vi "Main.vi"(11 "Module Admin":refnum<class "Delacor_lib_QMH_Module Admin.lvclass">) -> ()   [LabVIEW 2020, in "General UI.lvlib"]
doc: "This template is based off of the Queued Message Handler design pattern and the Queued Message Handler project template that ships with LabVIEW.\n\nThe main difference is that the queue is private to this module and communication between modules is performed via Broadcast and Request events.\n\nRequest events are wrapped in public API methods and are handled in the Event Handling Loop (EHL) of this VI. Any module can register for Broadcast events sent by this module. The EHL generates messages based on user interface actions.\n\nThe Message Handling Loop (MHL) processes messages generated by the EHL, or by other messages. The messages are string values, so new messages can be added easily to the Message Cases case structure in the MHL. Each message cluster can also provide an optional value for Message Data, which is a variant that can be converted to whatever message-specific data is required.\n_____\nBased on Delacor QMH Project Template 5.0.0.82."
uses:
  General UI.lvlib
  <vilib>/Delacor/Delacor QMH/Libraries/Module Admin_class/Delacor_lib_QMH_Module Admin.lvclass
  Module Data--cluster.ctl
  Stop Argument--cluster.ctl
  <vilib>/Delacor/Delacor QMH/Libraries/Message Queue_class/Delacor_lib_QMH_Message Queue.lvclass/Delacor_lib_QMH_Message Queue.ctl
  <vilib>/Delacor/Delacor QMH/Libraries/Module Admin_class/Delacor_lib_QMH_Module Admin.lvclass/Delacor_lib_QMH_Module Admin.ctl
  <vilib>/Delacor/Delacor QMH/Libraries/Message Queue_class/Delacor_lib_QMH_Enqueue Message (Single).vi
  <vilib>/Delacor/Delacor QMH/Libraries/Module Admin_class/Delacor_lib_QMH_Get External Launch.vi
  <vilib>/Utility/error.llb/Error Cluster From Error Code.vi
  <vilib>/ErrorRing/Error Ring.xnode
  <vilib>/Delacor/Delacor QMH/Libraries/Message Queue_class/Delacor_lib_QMH_Message Queue.lvclass
  Money Control Pane/Money Control Pane.lvlib
  Product Selecting Pane/Product Selecting Pane.lvlib
  Message Pane/Message Pane.lvlib
panel:
  out "error out":errorcluster
  in  "Exit":bool
  in  "Settings":bool
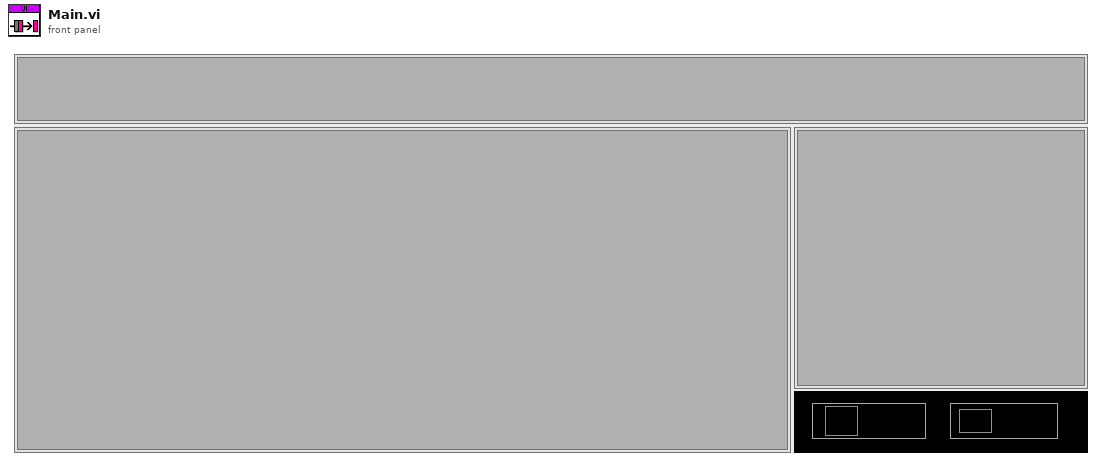
[diagram p1: front panel]
types:
  T1 = typedef "General UI.lvlib/Request Events--cluster.ctl" = cluster{"Stop Module":refnum<user-event>, "Show Panel":refnum<user-event>, "Hide Panel":refnum<user-event>, "Get Module Execution Status":refnum<user-event>, "Show Diagram":refnum<user-event>}
  T2 = typedef "Money Control Pane.lvlib/Broadcast Events--cluster.ctl" = cluster{"Module Did Init":refnum<user-event>, "Status Updated":refnum<user-event>, "Error Reported":refnum<user-event>, "Module Did Stop":refnum<user-event>, "Update Module Execution Status":refnum<user-event>}
  T3 = typedef "Product Selecting Pane.lvlib/Broadcast Events--cluster.ctl" = cluster{"Module Did Init":refnum<user-event>, "Status Updated":refnum<user-event>, "Error Reported":refnum<user-event>, "Module Did Stop":refnum<user-event>, "Update Module Execution Status":refnum<user-event>}
  T4 = typedef "Message Pane.lvlib/Broadcast Events--cluster.ctl" = cluster{"Module Did Init":refnum<user-event>, "Status Updated":refnum<user-event>, "Error Reported":refnum<user-event>, "Module Did Stop":refnum<user-event>, "Update Module Execution Status":refnum<user-event>}
  T5 = typedef "General UI.lvlib/Module Data--cluster.ctl" = cluster{"Status":string}
  T6 = enum32{"invalid lock state", "Not Locked", "Locked (No Password)", "Password-protected"}
  T7 = typedef "General UI.lvlib/Stop Argument--cluster.ctl" = cluster{"Origin":string, "Exit via Stop Module Req?":bool, "Wait for Module to stop?":bool}
  T8 = enum32{"Invalid", "Standard", "Closed", "Hidden", "Minimized", "Maximized"}
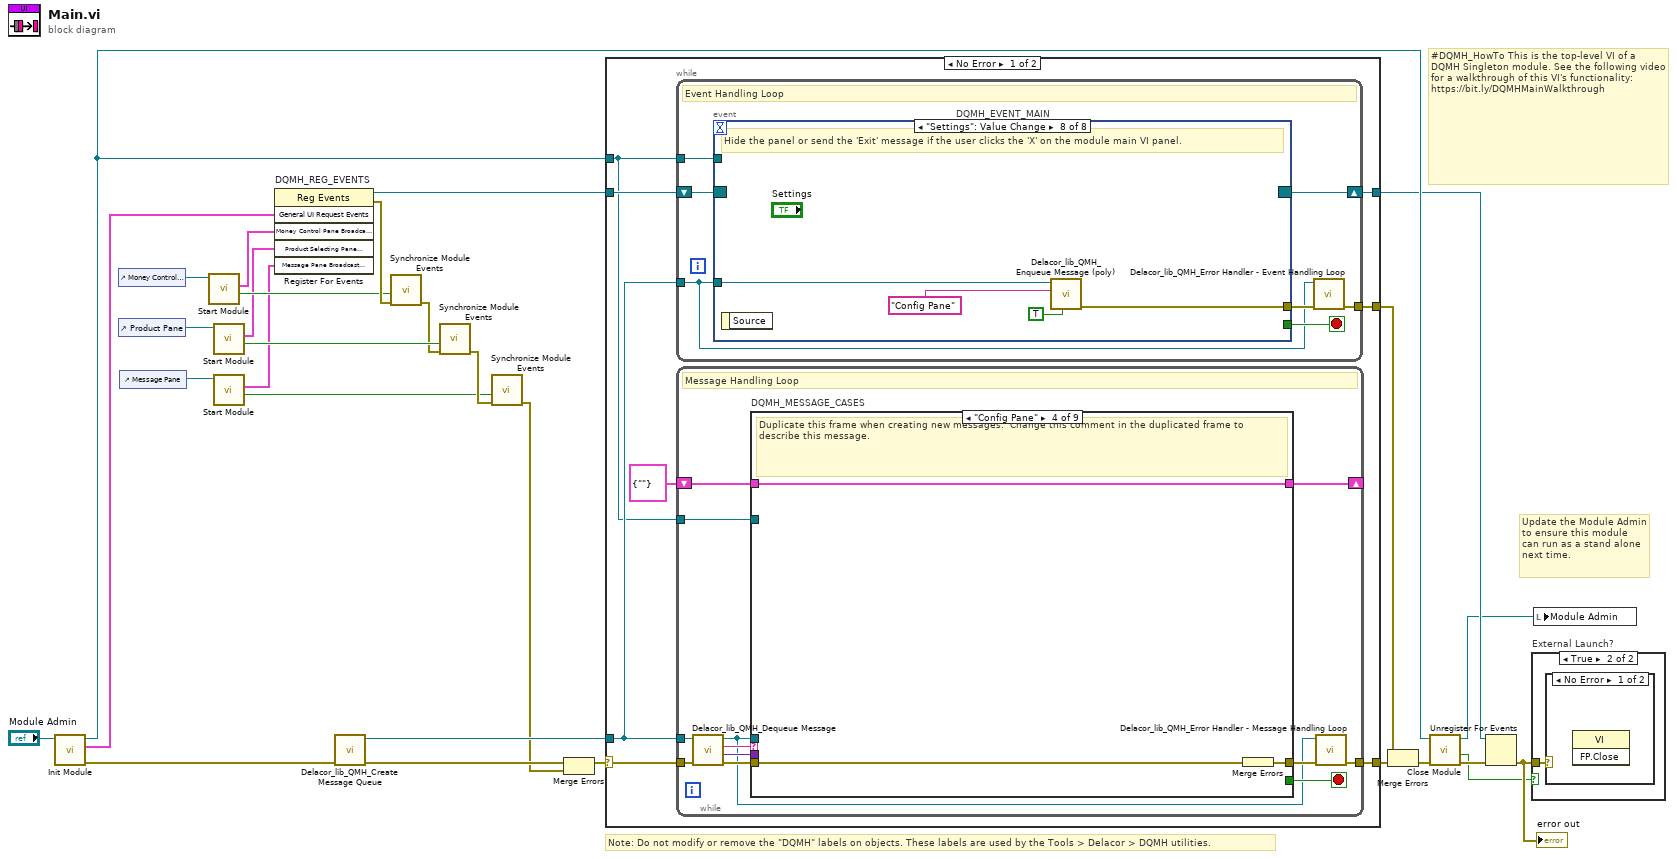
[diagram p0: block diagram]
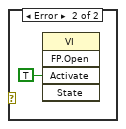
[diagram p3: hidden frame]
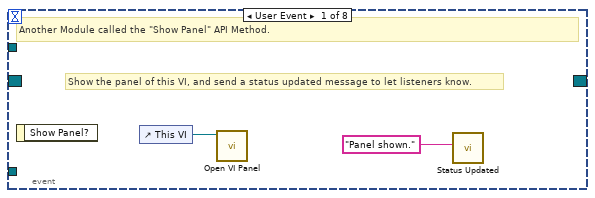
[diagram p4: hidden frame]
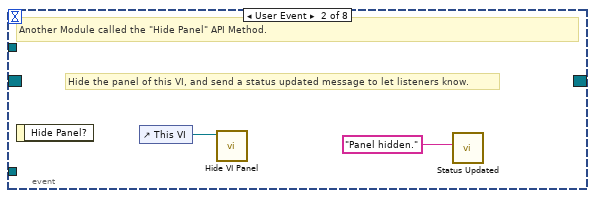
[diagram p5: hidden frame]
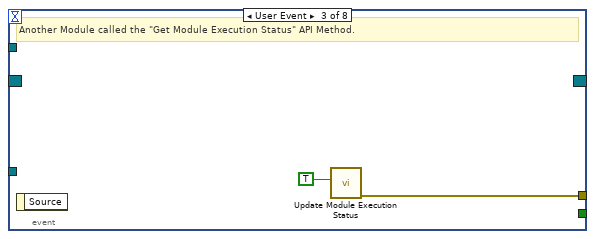
[diagram p6: hidden frame]
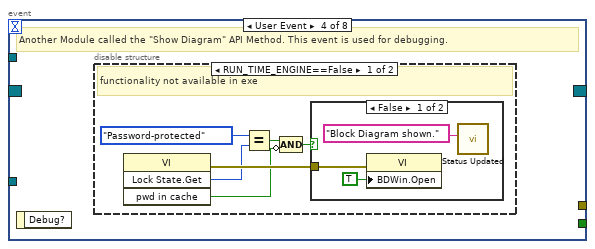
[diagram p7: hidden frame]
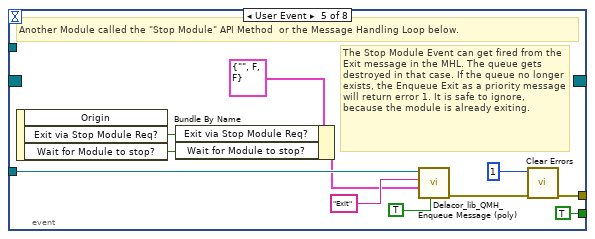
[diagram p10: hidden frame]
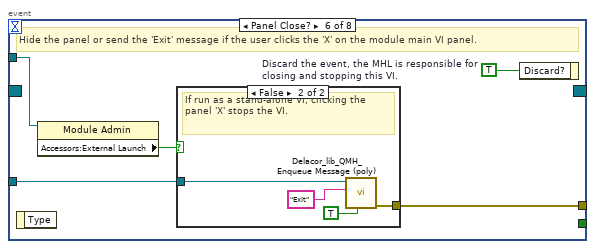
[diagram p11: hidden frame]
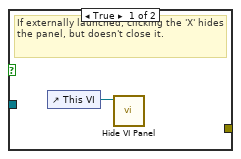
[diagram p12: hidden frame]
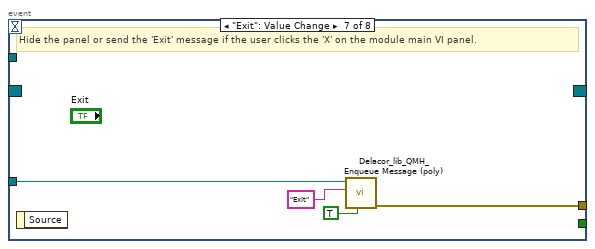
[diagram p13: hidden frame]
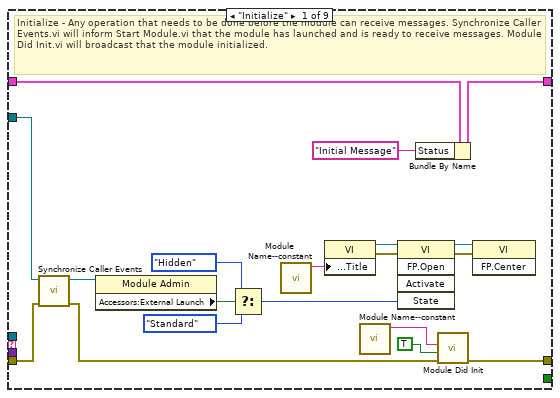
[diagram p14: hidden frame]
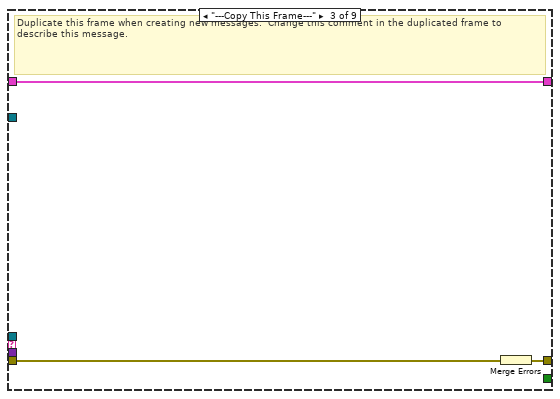
[diagram p16: hidden frame]
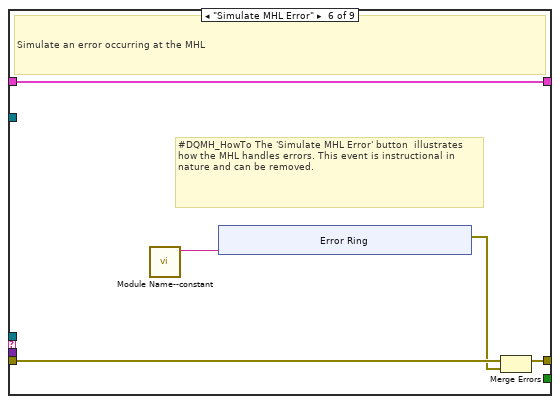
[diagram p18: hidden frame]
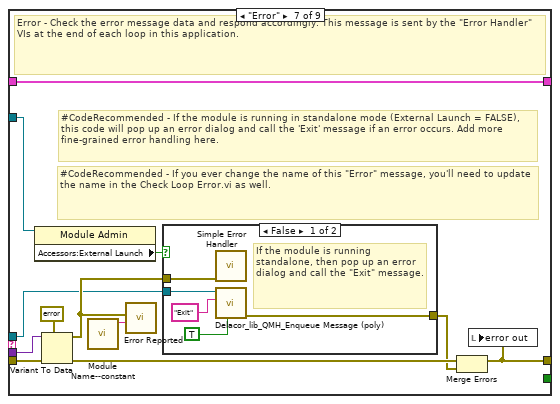
[diagram p19: hidden frame]
diagram:
  # "#DQMH_HowTo This is the top-level VI of a DQMH Singleton module. See the following video for a walkthrough of this VI's functionality: https://bit.ly/DQMHMainWalkthrough"
  # "Note: Do not modify or remove the \"DQMH\" labels on objects. These labels are used by the Tools > Delacor > DQMH utilities."
  # "Update the Module Admin to ensure this module can run as a stand alone next time."
  n1 = call "Init Module.vi"("Singleton Module Admin in"="Module Admin") -> ("error out"=w28:errorcluster, "General UI Request Events"=w18:T1, "Singleton Module Admin out"=w21:refnum<class "Delacor_lib_QMH_Module Admin.lvclass">)  [unwired: 8 in]
  n2 = control-ref of="Money Control Pane"() -> (w13:refnum<vi>)
  n3 = control-ref of="Product Pane"() -> (w9:refnum<vi>)
  n4 = control-ref of="Message Pane"() -> (w5:refnum<vi>)
  n5 = call "Start Module.vi"("MCP Sub Panel"=w13) -> ("Wait for Event Sync?"=w10:bool, "Money Control Pane Broadcast Events"=w12:T2)  [unwired: 7 in, 2 out]
  n6 = call "Start Module.vi"("Sub Panel"=w9) -> ("Wait for Event Sync?"=w8:bool, "Product Selecting Pane Broadcast Events"=w7:T3)  [unwired: 7 in, 2 out]
  n7 = call "Start Module.vi"("Sub Panel"=w5) -> ("Wait for Event Sync?"=w2:bool, "Message Pane Broadcast Events"=w1:T4)  [unwired: 7 in, 2 out]
  n8 = register-events "DQMH_REG_EVENTS"(w18, w12, w7, w1) -> (reference out=w19:refnum<event-registration>, error out=w11:errorcluster)  [unwired: 2 in]
  n9 = call <vilib>:"Delacor_lib_QMH_Create Message Queue.vi"("error in (no error)"=w28) -> ("error out"=w23:errorcluster, "Message Queue"=w17:refnum<class "Delacor_lib_QMH_Message Queue.lvclass">)  [unwired: 9 in]
  n10 = call "Synchronize Module Events.vi"("error in (no error)"=w11, "Wait for Event Sync?"=w10) -> ("error out"=w6:errorcluster)  [unwired: 9 in]
  n11 = call "Synchronize Module Events.vi"("error in (no error)"=w6, "Wait for Event Sync?"=w8) -> ("error out"=w4:errorcluster)  [unwired: 9 in]
  n12 = call "Synchronize Module Events.vi"("error in (no error)"=w4, "Wait for Event Sync?"=w2) -> ("error out"=w3:errorcluster)  [unwired: 9 in]
  n13 = Merge Errors(w23, w3) -> (w22:errorcluster)
  n14 = case shown="No Error" w22 {
    selector: w22 -> [w35 w190]
    tunnel: [w37 w189] -> w29
    tunnel: [w34 w195] -> w20
    tunnel: w19 -> [w32 w195]
    tunnel: w17 -> [w31 w188]
    tunnel: [w36 _] -> w26
    tunnel: w21 -> [w30 w191]
    frame No Error {
      n15 = while {
        tunnel: w31 -> [w38]
        shift-right: [w41] -> w34
        shift-left: w32 -> [w42]
        tunnel: [w43] -> w36
        tunnel: w30 -> [w39]
        stop <- w40 stop-if-true
        # "Event Handling Loop"
        n16 = event "DQMH_EVENT_MAIN" shown="[7] \"Settings\": Value Change" {
          selector: w42 -> [_ _ _ _ _ _ _ _]
          dyn-events: [_ _ _ _ _ _ _ _] -> w41
          timeout: _ -> [_ _ _ _ _ _ _ _]
          tunnel: [_ _ _ _ TRUE ("Discard?") _ _ _] -> w40
          tunnel: w38 -> [_ _ _ _ w66 w73 w83 w87]
          tunnel: [_ _ w50 _ w69 w75 w84 w88] -> w44
          tunnel: w39 -> [_ _ _ _ _ w72 _ _]
          event User Event {
            # "Show the panel of this VI, and send a status updated message to let listeners know."
            # "Another Module called the \"Show Panel\" API Method."
            n17 = event-data() -> ()  [unwired: 1 in, 1 out]
            n18 = control-ref of="This VI"() -> (w46:refnum<vi>)
            n19 = call "Open VI Panel.vi"("VI"=w46) -> ()  [unwired: 10 in, 1 out]
            n20 = call "Status Updated.vi"("Status"="Panel shown." ("format string")) -> ()  [unwired: 10 in, 1 out]
          }
          event User Event {
            # "Hide the panel of this VI, and send a status updated message to let listeners know."
            # "Another Module called the \"Hide Panel\" API Method."
            n21 = event-data() -> ()  [unwired: 1 in, 1 out]
            n22 = control-ref of="This VI"() -> (w48:refnum<vi>)
            n23 = call "Hide VI Panel.vi"("VI"=w48) -> ()  [unwired: 10 in, 1 out]
            n24 = call "Status Updated.vi"("Status"="Panel hidden." ("format string")) -> ()  [unwired: 10 in, 1 out]
          }
          event User Event {
            # "Another Module called the \"Get Module Execution Status\" API Method."
            n25 = event-data() -> ()  [unwired: 1 in, 1 out]
            n26 = call "Update Module Execution Status.vi"("Running?"=TRUE) -> ("error out"=w50:errorcluster)  [unwired: 10 in]
          }
          event User Event {
            # "Another Module called the \"Show Diagram\" API Method. This event is used for debugging."
            n27 = event-data() -> ()  [unwired: 1 in, 1 out]
            n28 = disable-structure shown="RUN_TIME_ENGINE==False" {
              frame condition #0 (active) {
                # "functionality not available in exe"
                n29 = invoke class="VI" method="Lock State.Get"() -> (error out=w56:errorcluster, "Get Lock State"=w55:T6, "pwd in cache"=w52:bool)  [unwired: 4 in, 1 out]
                n30 = Equal?(x=T6."Password-protected", y=w55) -> (x = y?=w53:bool)
                n31 = Compound Arithmetic op=AND(w53, invert w52) -> (w51:bool)
                n32 = case shown="False" w51 {
                  tunnel: w56 -> [w59 _]
                  frame False {
                    n33 = property class="VI"(error in=w59, "BDWin.Open"=TRUE ("Block Diagram Window:Open")) -> ()  [unwired: 1 in, 2 out]
                    n34 = call "Status Updated.vi"("Status"="Block Diagram shown." ("format string")) -> ()  [unwired: 10 in, 1 out]
                  }
                  frame True {
                    # "Password-protected VI, and the password is not in the cache. Do not show the diagram."
                  }
                }
              }
              frame condition #1 {
              }
            }
          }
          event User Event {
            # "The Stop Module Event can get fired from the Exit message in the MHL. The queue gets destroyed in that case. If the queue no longer exists, the Enqueue Exit as a priority message will return error 1. It is safe to ignore, because the module is already exiting."
            # "Another Module called the \"Stop Module\" API Method  or the Message Handling Loop below."
            n35 = event-data() -> ("Exit via Stop Module Req?"=w62:bool, "Wait for Module to stop?"=w61:bool)  [unwired: 1 in, 1 out]
            n36 = Bundle By Name(cluster=T7 {"Origin"="", "Exit via Stop Module Req?"=FALSE, "Wait for Module to stop?"=FALSE} ("Stop Argument"), "Exit via Stop Module Req?"=w62, "Wait for Module to stop?"=w61) -> (w60:T7)
            n37 = call-poly <vilib>:"Delacor_lib_QMH_Enqueue Message (poly).vi"("Priority Message? (F)"=TRUE, "Message Data"=w60, "Message"="Exit", "Message Queue in"=w66) -> ("error out"=w70:errorcluster)  [unwired: 6 in, 1 out]
            n38 = call <vilib>:"Clear Errors.vi"("error in (no error)"=w70, "specific error code to clear (0: all)"=1) -> ("error out"=w69:errorcluster)  [unwired: 4 in, 1 out]
          }
          event Panel Close? {
            w74 = TRUE  # Discard the event, the MHL is responsible for closing and stopping this VI.
            # "Hide the panel or send the 'Exit' message if the user clicks the 'X' on the module main VI panel."
            n39 = event-data() -> ()  [unwired: 1 in, 1 out]
            n40 = property class="Module Admin"(reference=w72) -> ("Accessors:External Launch"=w71:bool)  [unwired: 1 in, 2 out]
            n41 = case shown="False" w71 {
              tunnel: w73 -> [_ w79]
              tunnel: [_ w80] -> w75
              frame True {
                # "If externally launched, clicking the 'X' hides the panel, but doesn't close it."
                n42 = control-ref of="This VI"() -> (w76:refnum<vi>)
                n43 = call "Hide VI Panel.vi"("VI"=w76) -> ()  [unwired: 10 in, 1 out]
              }
              frame False {
                # "If run as a stand-alone VI, clicking the panel 'X' stops the VI."
                n44 = call-poly <vilib>:"Delacor_lib_QMH_Enqueue Message (poly).vi"("Priority Message? (F)"=TRUE, "Message"="Exit", "Message Queue in"=w79) -> ("error out"=w80:errorcluster)  [unwired: 7 in, 1 out]
              }
            }
            n45 = event-data("Discard?"=w74) -> ()  [unwired: 1 in, 1 out]
          }
          event "Exit": Value Change {
            # "Hide the panel or send the 'Exit' message if the user clicks the 'X' on the module main VI panel."
            n46 = event-data() -> ()  [unwired: 1 in, 1 out]
            n47 = call-poly <vilib>:"Delacor_lib_QMH_Enqueue Message (poly).vi"("Priority Message? (F)"=TRUE, "Message"="Exit", "Message Queue in"=w83) -> ("error out"=w84:errorcluster)  [unwired: 7 in, 1 out]
          }
          event "Settings": Value Change {
            # "Hide the panel or send the 'Exit' message if the user clicks the 'X' on the module main VI panel."
            n48 = event-data() -> ()  [unwired: 1 in, 1 out]
            n49 = call-poly <vilib>:"Delacor_lib_QMH_Enqueue Message (poly).vi"("Priority Message? (F)"=TRUE, "Message"="Config Pane", "Message Queue in"=w87) -> ("error out"=w88:errorcluster)  [unwired: 7 in, 1 out]
          }
        }
        n50 = call-dynamic "Delacor_lib_QMH_Error Handler - Event Handling Loop.vi"("error in (no error)"=w44, "Message Queue in"=w38) -> ("dup error in"=w43:errorcluster)  [unwired: 8 in, 1 out]
      }
      n51 = while {
        tunnel: w31 -> [w91]
        shift-right: [w95] -> _
        shift-left: T5 {"Status"=""} ("Data Cluster") -> [w96]
        tunnel: w35 -> [w99]
        tunnel: [w97] -> w37
        tunnel: w30 -> [w89]
        stop <- w94 stop-if-true
        # "Message Handling Loop"
        n52 = call-dynamic "Delacor_lib_QMH_Dequeue Message.vi"("error in (no error)"=w99, "Message Queue in"=w91) -> ("error out"=w98:errorcluster, "Message Data"=w92:variant, "Message"=w93:string, "Message Queue out"=w90:refnum<class "Delacor_lib_QMH_Message Queue.lvclass">)  [unwired: 6 in]
        n53 = case "DQMH_MESSAGE_CASES" shown="\"Config Pane\"" w93 {
          selector: w93 -> [_ _ _ _ _ _ _ _ w175]
          tunnel: w90 -> [_ _ _ _ _ _ w145 w167 _]
          tunnel: w98 -> [w117 w121 w124 w127 w129 w134 w152 w173 w177]
          tunnel: [w115 w121 w123 w126 w129 w133 w148 w170 w178] -> w100
          tunnel: w96 -> [w106 w120 w122 w125 w128 w131 w147 w166 w176]
          tunnel: [w105 w120 w122 w125 w128 w131 w147 w166 w176] -> w95
          tunnel: [_ _ _ _ _ _ _ w165 _] -> w94
          tunnel: w92 -> [_ _ _ _ _ _ w146 w164 _]
          tunnel: w89 -> [w107 _ _ _ _ _ w144 w159 _]
          frame "Initialize" {
            # "Initialize - Any operation that needs to be done before the module can receive messages. Synchronize Caller Events.vi will inform Start Module.vi that the module has launched and is ready to receive messages. Module Did Init.vi will broadcast that the module initialized."
            n54 = call "Synchronize Caller Events.vi"("error in (no error)"=w117, "Singleton Module Admin in"=w107) -> ("error out"=w116:errorcluster, "Singleton Module Admin out"=w102:refnum<class "Delacor_lib_QMH_Module Admin.lvclass">)  [unwired: 8 in]
            n55 = property class="Module Admin"(reference=w102) -> ("Accessors:External Launch"=w111:bool)  [unwired: 1 in, 2 out]
            n56 = Select(t=T8."Hidden" ("State"), s=w111, f=T8."Standard" ("State")) -> (s? t:f=w108:T8)
            n57 = call "Module Name--constant.vi"() -> ("Module Name"=w114:string)  [unwired: 11 in]
            n58 = property class="VI"("Front Panel.Title"=w114) -> (reference out=w113:refnum<vi>, error out=w119:errorcluster)  [unwired: 2 in]
            n59 = call "Module Name--constant.vi"() -> ("Module Name"=w103:string)  [unwired: 11 in]
            n60 = invoke class="VI" method="FP.Open"(reference=w113, error in=w119, "State"=w108) -> (reference out=w112:refnum<vi>, error out=w118:errorcluster)  [unwired: 2 in, 3 out]
            n61 = Bundle By Name(cluster=w106, "Status"="Initial Message" ("Initial Message")) -> (w105:T5)
            n62 = call "Module Did Init.vi"("error in (no error)"=w116, "Initialized?"=TRUE, "Origin"=w103) -> ("error out"=w115:errorcluster)  [unwired: 8 in]
            n63 = invoke class="VI" method="FP.Center"(reference=w112, error in=w118) -> ()  [unwired: 1 in, 3 out]
          }
          frame "--- Module Specific ---" {
            # "Separator -- The following cases handle messages specific to this Module."
          }
          frame "---Copy This Frame---" {
            # "Duplicate this frame when creating new messages.  Change this comment in the duplicated frame to describe this message."
            n64 = Merge Errors(w124) -> (w123:errorcluster)
          }
          frame "Config Pane" {
            # "Duplicate this frame when creating new messages.  Change this comment in the duplicated frame to describe this message."
            n65 = Merge Errors(w127) -> (w126:errorcluster)
          }
          frame "--- Exit and Error Handling---" {
            # "Separator - The following cases handle errors and exit messages."
          }
          frame "Simulate MHL Error" {
            # "#DQMH_HowTo The 'Simulate MHL Error' button  illustrates how the MHL handles errors. This event is instructional in nature and can be removed."
            # "Simulate an error occurring at the MHL"
            n66 = call "Module Name--constant.vi"() -> ("Module Name"=w130:string)  [unwired: 11 in]
            n67 = xnode "Error Ring"("parameter 0"=w130) -> ("error out"=w132:errorcluster)
            n68 = Merge Errors(w134, w132) -> (w133:errorcluster)
          }
          frame "Error" {
            # "#CodeRecommended - If you ever change the name of this \"Error\" message, you'll need to update the name in the Check Loop Error.vi as well."
            # "#CodeRecommended - If the module is running in standalone mode (External Launch = FALSE), this code will pop up an error dialog and call the 'Exit' message if an error occurs. Add more fine-grained error handling here."
            # "Error - Check the error message data and respond accordingly. This message is sent by the \"Error Handler\" VIs at the end of each loop in this application."
            n69 = property class="Module Admin"(reference=w144) -> ("Accessors:External Launch"=w143:bool)  [unwired: 1 in, 2 out]
            n70 = Variant To Data(error in=w152, type=errorcluster {"status"=FALSE, "code"=0, "source"=""} ("error constant"), Variant=w146) -> (data=w153:errorcluster, error out=w150:errorcluster)
            n71 = call "Module Name--constant.vi"() -> ("Module Name"=w142:string)  [unwired: 11 in]
            n72 = call "Error Reported.vi"("Additional Information"=w142, "Error"=w153) -> ()  [unwired: 9 in, 1 out]
            n73 = case shown="False" w143 {
              tunnel: [w158 _] -> w149
              tunnel: w145 -> [w156 _]
              tunnel: w153 -> [w157 _]
              frame False {
                # "If the module is running standalone, then pop up an error dialog and call the \"Exit\" message."
                n74 = call <vilib>:"Simple Error Handler.vi"("error in (no error)"=w157) -> ()  [unwired: 4 in, 5 out]
                n75 = call-poly <vilib>:"Delacor_lib_QMH_Enqueue Message (poly).vi"("Priority Message? (F)"=TRUE, "Message"="Exit", "Message Queue in"=w156) -> ("error out"=w158:errorcluster)  [unwired: 7 in, 1 out]
              }
              frame True {
                # "If the module was launched externally, calling the Error Reported broadcast VI is the only action performed by the \"Error\" message. The module's caller can then process the error appropriately."
              }
            }
            n76 = Merge Errors(w150, w149) -> (w148:errorcluster)
            n77 = local write "error out"(w148) -> ()
          }
          frame "Exit" {
            w163 = 91  # 91: not all Exit messages will have an argument
            w165 = TRUE  # Stop the VI
            # "Release the message queue reference"
            # "#CodeNeeded - Add any required cleanup code here"
            # "Exit - Exit the application."
            n78 = Variant To Data(error in=w173, type=T7 {"Origin"="", "Exit via Stop Module Req?"=FALSE, "Wait for Module to stop?"=FALSE} ("Stop Argument"), Variant=w164) -> (data=w161:T7, error out=w169:errorcluster)
            n79 = call <vilib>:"Clear Errors.vi"("error in (no error)"=w169, "specific error code to clear (0: all)"=w163) -> ("error out"=w172:errorcluster)  [unwired: 4 in, 1 out]
            n80 = control-ref of="This VI"() -> (w160:refnum<vi>)
            n81 = call-dynamic "Delacor_lib_QMH_Release Message Queue.vi"("error in (no error)"=w172, "Message Queue"=w167) -> ("error out"=w171:errorcluster)  [unwired: 9 in]
            n82 = call "Handle Exit.vi"("Stop Argument"=w161, "Admin in"=w159, "VI reference"=w160) -> ("error out"=w168:errorcluster)  [unwired: 7 in, 1 out]
            n83 = Merge Errors(w171, w168) -> (w170:errorcluster)
            n84 = call "Stop Module.vi"() -> ()  [unwired: 11 in, 1 out]
            n85 = call "Stop Module.vi"() -> ()  [unwired: 11 in, 1 out]
            n86 = call "Stop Module.vi"() -> ()  [unwired: 11 in, 1 out]
          }
          frame Default {
            # "'Default' case only runs if there is a message that isn't defined in any of the other cases.  Output a programming error."
            n87 = call "Module Name--constant.vi"() -> ("Module Name"=w174:string)  [unwired: 11 in]
            n88 = xnode "Error Ring"("parameter 0"=w175, "parameter 1"=w174) -> ("error out"=w179:errorcluster)
            n89 = Merge Errors(w177, w179) -> (w178:errorcluster)
          }
        }
        n90 = call-dynamic "Delacor_lib_QMH_Error Handler - Message Handling Loop.vi"("error in (no error)"=w100, "Message Queue in"=w90) -> ("dup error in"=w97:errorcluster)  [unwired: 8 in, 1 out]
      }
    }
    frame Error {
      # "Synchronize Caller Events.vi will inform Start Module.vi that the module has launched and will let the code calling Start Module.vi register for broadcasts and would permit the caller receive the broadcast that an error occurred at launch time."
      n91 = call-dynamic "Delacor_lib_QMH_Release Message Queue.vi"("error in (no error)"=w190, "Message Queue"=w188) -> ("error out"=w189:errorcluster)  [unwired: 9 in]
      n92 = call "Synchronize Caller Events.vi"("Singleton Module Admin in"=w191) -> ("error out"=w196:errorcluster)  [unwired: 9 in, 1 out]
      n93 = call "Module Name--constant.vi"() -> ("Module Name"=w194:string)  [unwired: 11 in]
      n94 = Format Into String(format string="An error occurred during initialization. %s is no longer running.", w194) -> (resulting string=w192:string)  [unwired: 2 in, 1 out]
      n95 = Merge Errors(w189, w196) -> (w197:errorcluster)
      n96 = call "Error Reported.vi"("Additional Information"=w192, "Error"=w197) -> ()  [unwired: 9 in, 1 out]
    }
  }
  n97 = Merge Errors(w26, w29) -> (w25:errorcluster)
  n98 = call "Close Module.vi"("error in (no error)"=w25, "Module Admin in"=w21) -> ("error out"=w27:errorcluster, "External Launch"=w14:bool, "Module Admin out"=w15:refnum<class "Delacor_lib_QMH_Module Admin.lvclass">)  [unwired: 7 in]
  n99 = Unregister For Events(event registration refnum=w20, error in=w27) -> (error out=w24:errorcluster)
  "error out" <- w24
  n100 = case "External Launch?" shown="True" w14 {
    tunnel: w24 -> [_ w198]
    frame False {
    }
    frame True {
      n101 = case shown="No Error" w198 {
        frame No Error {
          n102 = invoke class="VI" method="FP.Close"() -> ()  [unwired: 3 in, 3 out]
        }
        frame Error {
          n103 = invoke class="VI" method="FP.Open"("Activate"=TRUE ("Activate?")) -> ()  [unwired: 4 in, 5 out]
        }
      }
    }
  }
  n104 = local write "Module Admin"(w15) -> ()
